vi "Scale.vi"   [LabVIEW 2018, in "NI_AALBase.lvlib"]
doc: "Removes the <B>offset</B> of an input signal <B>X</B> and then scales the result so that the output sequence is in the range [-1:1]."
uses:
  NI_AALBase.lvlib
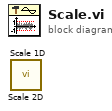
[diagram p0: block diagram]
diagram:
  n1 = call "Scale 2D.vi"() -> ()  [unwired: 1 in, 4 out]
  n2 = call "Scale 1D.vi"() -> ()  [unwired: 1 in, 4 out]
